vi "ReadgRPCDetails.vi"(8 "error in (no error)":errorcluster, 11 "MicronGRPCClient in":refnum<class "MicronGRPCClient.lvclass">) -> (0 "error out":errorcluster, 2 "gRPCDetails":T1, 3 "MicronGRPCClient out":refnum<class "MicronGRPCClient.lvclass">)   [LabVIEW 2019, in "MicronGRPCClient.lvclass"]
uses:
  MicronGRPCClient.lvclass
  Typedefs/gRPCDetails.ctl
  <vilib>/gRPC/LabVIEW gRPC Library/Shared/grpcId.ctl
  MicronGRPCClient.lvclass/MicronGRPCClient.ctl
  <vilib>/gRPC/LabVIEW gRPC Library/grpc-lvsupport-release.lvlib
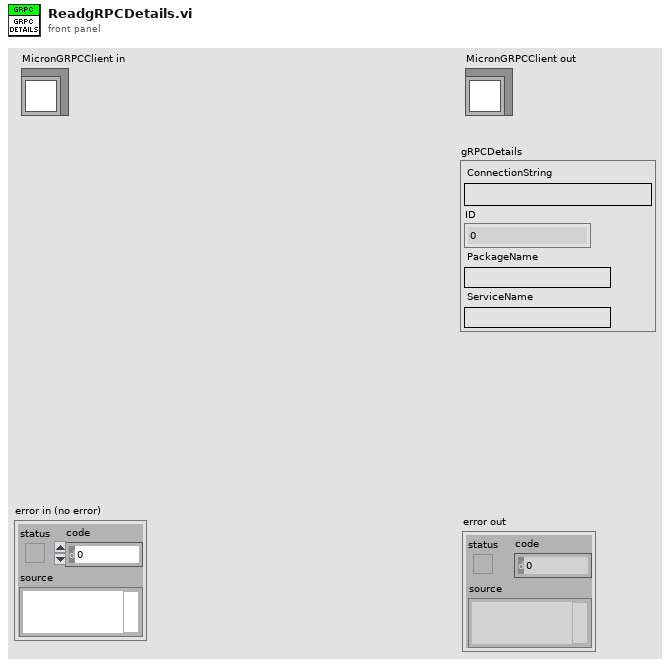
[diagram p1: front panel]
types:
  T1 = typedef "MicronGRPCClient.lvclass/gRPCDetails.ctl" = cluster{"ConnectionString":string, "ID":T2, "PackageName":string, "ServiceName":string}
  T2 = typedef "grpc-lvsupport-release.lvlib/grpcId.ctl" = u64
  T3 = typedef "MicronGRPCClient.lvclass/InternalCluster.ctl" = cluster{"ServiceDetails":T4, "gRPCDetails":T5}
  T4 = typedef "MicronClient.lvclass/ServiceDetails.ctl" = cluster{"MicronPath":path, "Network":string, "ServiceID":string, "Port":i32, "FullyQualifiedName":string, "UI":string, "Args":string, "Mode":string, "AutoRestartOnError?":bool, "Simulate?":bool}
  T5 = typedef "gRPCDetails.ctl" = cluster{"ConnectionString":string, "ID":T2, "PackageName":string, "ServiceName":string}
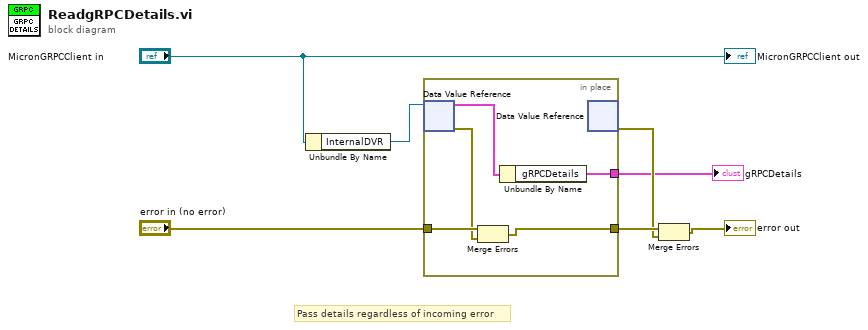
[diagram p0: block diagram]
diagram:
  # "Pass details regardless of incoming error"
  n1 = Unbundle By Name("MicronGRPCClient in") -> ("InternalDVR"=w4:refnum<data-value>)
  n2 = in-place {
    in-place-border: "error in (no error)" -> [w12]
    in-place-border: [w10] -> w3
    in-place-border: [w8] -> w1
    n3 = in-place-dvr #1(w4) -> (w9:T3, w11:errorcluster)
    n4 = Merge Errors(w12, w11) -> (w10:errorcluster)
    n5 = Unbundle By Name(w9) -> ("gRPCDetails"=w8:T5)
    n6 = in-place-dvr #1() -> (w2:errorcluster)  [unwired: 1 in, 1 out]
  }
  "gRPCDetails" <- w1
  n7 = Merge Errors(w3, w2) -> (→"error out":errorcluster)
  "MicronGRPCClient out" <- "MicronGRPCClient in"
